vi "LIST OBJECTS.vi"() -> ()   [LabVIEW 2018]
uses:
  Typedefs/key-value-type cluster.ctl
  demo/Implementations/Product-A.lvclass
  U:/modules/labview-orm/_Serializable Base Object/_ISerializable.lvclass
  <vilib>/addons/database/Connection.llb/DB Tools Open Connec (Path).vi
  <vilib>/addons/database/Connection.llb/Conn Execute.vi
  <vilib>/addons/database/Recordset.llb/Rec Fetch Recordset Data (R).vi
  <vilib>/addons/database/Recordset.llb/Rec Destroy - Connection.vi
  <vilib>/addons/database/NI_Database_API.lvlib
  Serializer/Serializer.lvclass
  ORM/LV-ORM.lvclass
panel:
  out "x-y 4":u32
  out "x-y 3":u32
  out "x-y 2":u32
  out "x-y":u32
  out "Numeric 2":u32
  out "Numeric":u32
  out "Array 2":refnum<class "Product-A.lvclass">[](array[class])
  out "Array 3":T1[][](array[typedef])
  out "key-value-type":T1[](array[typedef])
  out "error out":errorcluster
  in  "table":string="Product-A"
  out "Array":string[][](array[string])
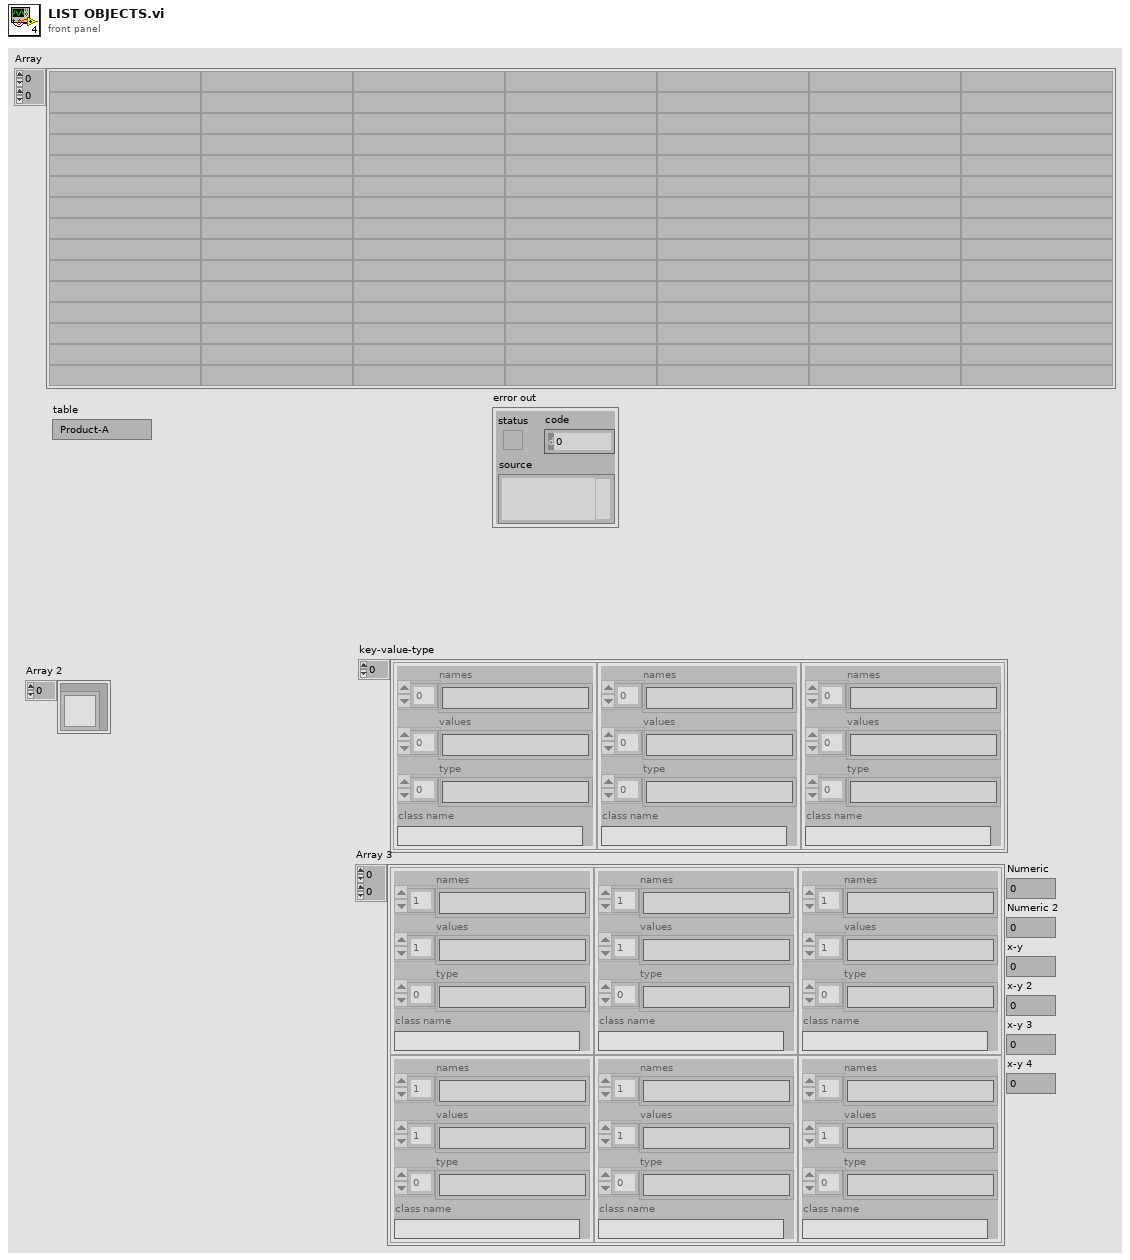
[diagram p1: front panel]
types:
  T1 = typedef "key-value-type cluster.ctl" = cluster{"names":string[], "values":string[], "type":string[], "class name":string}
  T2 = typedef "NI_Database_API.lvlib/Conn ObjectReference.ctl" = refnum<k1>
  T3 = typedef "NI_Database_API.lvlib/Rec ObjectReference.ctl" = refnum<k1>
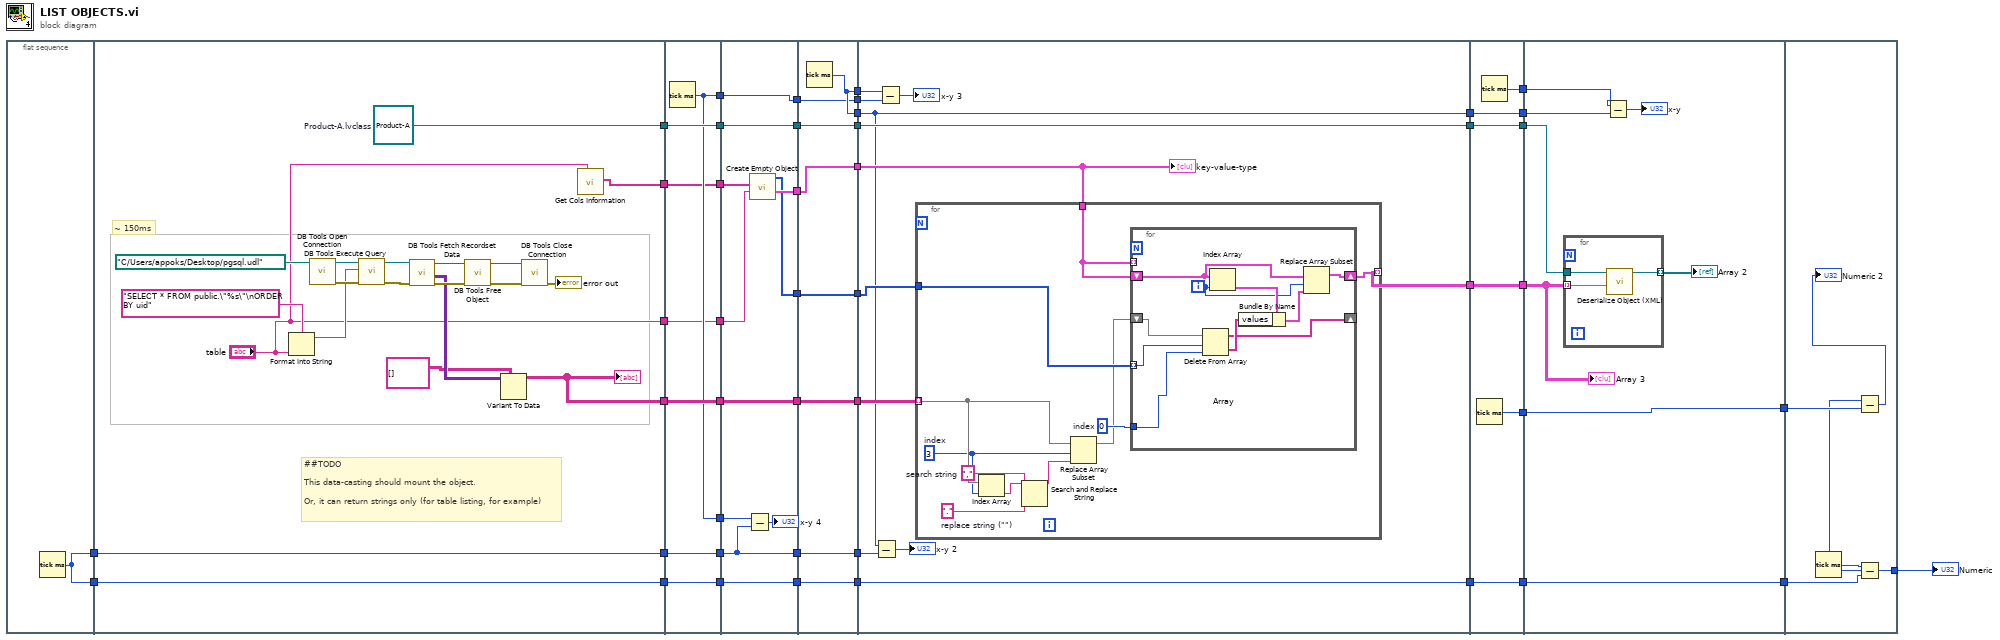
[diagram p0: block diagram]
diagram:
  n1 = flat-sequence {
    tunnel: [w46] -> w45
    tunnel: [w46] -> w25
    tunnel: [w52] -> w18
    tunnel: w45 -> [w52]
    tunnel: [w51] -> w16
    tunnel: [w50] -> w14
    tunnel: w25 -> [w49]
    tunnel: [w49] -> w12
    tunnel: ["table"] -> w3
    tunnel: [w48] -> w1
    tunnel: w18 -> [w73]
    tunnel: [w73] -> w17
    tunnel: w16 -> [w72]
    tunnel: [w72] -> w15
    tunnel: w14 -> [w71]
    tunnel: [w71] -> w13
    tunnel: w12 -> [w70]
    tunnel: [w70] -> w11
    tunnel: [w69] -> w10
    tunnel: [w69] -> w6
    tunnel: [w68] -> w4
    tunnel: w3 -> [w68]
    tunnel: [w67] -> w2
    tunnel: w1 -> [w67]
    tunnel: w17 -> [w84]
    tunnel: [w84] -> w23
    tunnel: w15 -> [w82]
    tunnel: [w82] -> w22
    tunnel: w13 -> [w83]
    tunnel: [w83] -> w21
    tunnel: [w75] -> w20
    tunnel: w11 -> [w79]
    tunnel: [w79] -> w19
    tunnel: w10 -> [w81]
    tunnel: [w81] -> w8
    tunnel: w6 -> [w80]
    tunnel: [w77] -> w5
    tunnel: w4 -> [w76]
    tunnel: w2 -> [w74]
    tunnel: w23 -> [w92]
    tunnel: [w92] -> w34
    tunnel: w22 -> [w91]
    tunnel: [w91] -> w33
    tunnel: [w85] -> w32
    tunnel: w21 -> [w90]
    tunnel: [w90] -> w31
    tunnel: w20 -> [w89]
    tunnel: [w89] -> w30
    tunnel: [w87] -> w28
    tunnel: w19 -> [w88]
    tunnel: [w88] -> w24
    tunnel: [w87] -> w9
    tunnel: w8 -> [w86]
    tunnel: [w86] -> w7
    tunnel: w5 -> [w85]
    tunnel: w34 -> [w104]
    tunnel: [w104] -> w37
    tunnel: [w99] -> w36
    tunnel: w33 -> [w103]
    tunnel: [w103] -> w35
    tunnel: w32 -> [w101]
    tunnel: w31 -> [w102]
    tunnel: w30 -> [w100]
    tunnel: w28 -> [w97]
    tunnel: [w97] -> w27
    tunnel: w24 -> [w98]
    tunnel: w9 -> [w95]
    tunnel: w7 -> [w94]
    tunnel: w37 -> [w131]
    tunnel: [w131] -> w41
    tunnel: w36 -> [w130]
    tunnel: [w130] -> w40
    tunnel: w35 -> [w129]
    tunnel: [w129] -> w39
    tunnel: [w128] -> w38
    tunnel: [w127] -> w29
    tunnel: w27 -> [w126]
    tunnel: [w126] -> w26
    tunnel: w41 -> [w139]
    tunnel: [w139] -> w43
    tunnel: w40 -> [w136]
    tunnel: w39 -> [w137]
    tunnel: [w135] -> w42
    tunnel: w38 -> [w135]
    tunnel: w29 -> [w134]
    tunnel: w26 -> [w133]
    tunnel: w43 -> [w147]
    tunnel: [w146] -> w44
    tunnel: w42 -> [w145]
    frame #0 {
      n2 = Tick Count (ms)() -> (millisecond timer value=w46:u32)
    }
    frame #1 {
      w51 = refnum<class "Product-A.lvclass"> refnum  # Product-A.lvclass
      # "~ 150ms"
      # "##TODO\n\nThis data-casting should mount the object.\n\nOr, it can return strings only (for table listing, for example)"
      n3 = Format Into String(format string="SELECT * FROM public.\"%s\"\nORDER BY uid", "table") -> (resulting string=w54:string)  [unwired: 2 in, 1 out]
      n4 = call-poly <vilib>:"DB Tools Open Connection.vi"("connection information"=path "C:/Users/appoks/Desktop/pgsql.udl") -> ("error out"=w59:errorcluster, "connection reference"=w58:T2)  [unwired: 7 in]
      n5 = call-poly <vilib>:"DB Tools Execute Query.vi"("error in (no error)"=w59, "SQL query"=w54, "connection reference"=w58) -> ("error out"=w62:errorcluster, "recordset reference"=w63:T3)  [unwired: 5 in]
      n6 = call-poly <vilib>:"DB Tools Fetch Recordset Data.vi"("error in (no error)"=w62, "recordset reference"=w63) -> ("error out"=w60:errorcluster, "recordset data"=w57:variant[][], "recordset reference out"=w61:T3)  [unwired: 3 in]
      n7 = call-poly <vilib>:"DB Tools Free Object.vi"("error in (no error)"=w60, "recordset reference"=w61) -> ("error out"=w64:errorcluster, "connection reference"=w65:T2)  [unwired: 8 in]
      n8 = Variant To Data(type=string[][] [], Variant=w57) -> (data=w50:string[][])  [unwired: 1 in, 1 out]
      "Array" <- w50
      n9 = call <vilib>:"DB Tools Close Connection.vi"("error in (no error)"=w64, "connection reference"=w65) -> ("error out"=→"error out":errorcluster)  [unwired: 5 in]
      n10 = call "Get Cols Information.vi"("Table Name"="table") -> ("columns data type"=w48:string[])  [unwired: 7 in, 3 out]
    }
    frame #2 {
      n11 = Tick Count (ms)() -> (millisecond timer value=w69:u32)
    }
    frame #3 {
      n12 = Subtract(x=w80, y=w79) -> (x-y=→"x-y 4":u32)
      n13 = call "Create Empty Object.vi"("Table Name"=w76, "columns data type"=w74) -> ("Array 3"=w77:T1[], "elements by level"=w75:i32[])  [unwired: 8 in]
    }
    frame #4 {
      n14 = Tick Count (ms)() -> (millisecond timer value=w87:u32)
    }
    frame #5 {
      n15 = Subtract(x=w97, y=w98) -> (x-y=→"x-y 2":u32)
      n16 = Subtract(x=w95, y=w94) -> (x-y=→"x-y 3":u32)
      n17 = for {
        tunnel: w102 -> [w110] mode=indexing
        tunnel: w101 -> [w115]
        tunnel: w100 -> [w114]
        tunnel: [w113] -> w99 mode=indexing
        w106 = "."  # replace string ("")
        w107 = ","  # search string
        w109 = 3  # index
        w112 = 0  # index
        n18 = Index Array(array=w110, index=w109) -> (element=w108:string)
        n19 = Search and Replace String(input string=w108, search string=w107, replace string=w106) -> (result string=w105:string)  [unwired: 5 in, 3 out]
        n20 = Replace Array Subset(array=w110, new element=w105, index=w109) -> (w111:string[])
        n21 = for {
          shift-right: [w120] -> w113
          shift-left: w115 -> [w121]
          tunnel: w115 -> [_] mode=indexing
          shift-right: [w122] -> _
          shift-left: w111 -> [w124]
          tunnel: w112 -> [w117]
          tunnel: w114 -> [w116] mode=indexing
          i -> [w118]
          n22 = Delete From Array(array=w124, length=w116, index=w117) -> (deleted portion=w123:string[], array with subset deleted=w122:string[])
          n23 = Index Array(array=w121, index=w118) -> (element=w125:T1)
          n24 = Bundle By Name(cluster=w125, "values"=w123) -> (w119:T1)
          n25 = Replace Array Subset(array=w121, new element=w119, index=w118) -> (w120:T1[])
        }
      }
      "key-value-type" <- w101
    }
    frame #6 {
      n26 = Tick Count (ms)() -> (millisecond timer value=w128:u32)
      n27 = Tick Count (ms)() -> (millisecond timer value=w127:u32)
    }
    frame #7 {
      n28 = for {
        tunnel: w136 -> [w140] mode=indexing
        tunnel: w137 -> [w142]
        tunnel: [w141] -> w138 mode=indexing
        n29 = call "Deserialize Object (XML).vi"("key-value-type in"=w140, "object type"=w142) -> ("object out"=w141:refnum<class "Product-A.lvclass">)  [unwired: 8 in, 1 out]
      }
      "Array 2" <- w138
      n30 = Subtract(x=w134, y=w133) -> (x-y=→"x-y":u32)
      "Array 3" <- w136
    }
    frame #8 {
      n31 = Tick Count (ms)() -> (millisecond timer value=w144:u32)
      n32 = Subtract(x=w144, y=w145) -> (x-y=→"Numeric 2":u32)
      n33 = Subtract(x=w144, y=w147) -> (x-y=w146:u32)
    }
  }
  "Numeric" <- w44
